vi "Write_CSV_date_time.vi"() -> ()   [LabVIEW 2015]
uses:
  <vilib>/Utility/file.llb/Write Delimited Spreadsheet (DBL).vi
  <vilib>/Utility/file.llb/Write To Spreadsheet File (string).vi
panel:
  in  "Values to Write":i32=20
  out "Array":string[](array[string])
  out "appended array":string[][](array[string])
  in  "# No Channel":i32=5
  in  "stop":bool
  in  "Header Info":string[][](table)=[["Test Name", "Operator", "UUT"], ["Voltage Test", "Nigel", "AAA123"]]
  in  "File Name":path=path "C:/Documents and Settings/husmith/Desktop/CSVdata.csv"
  in  "Channel Names":string[](array[string])=["Channel 1", "Channel 2", "Channel 3", "Channel 4", "Channel 5"]
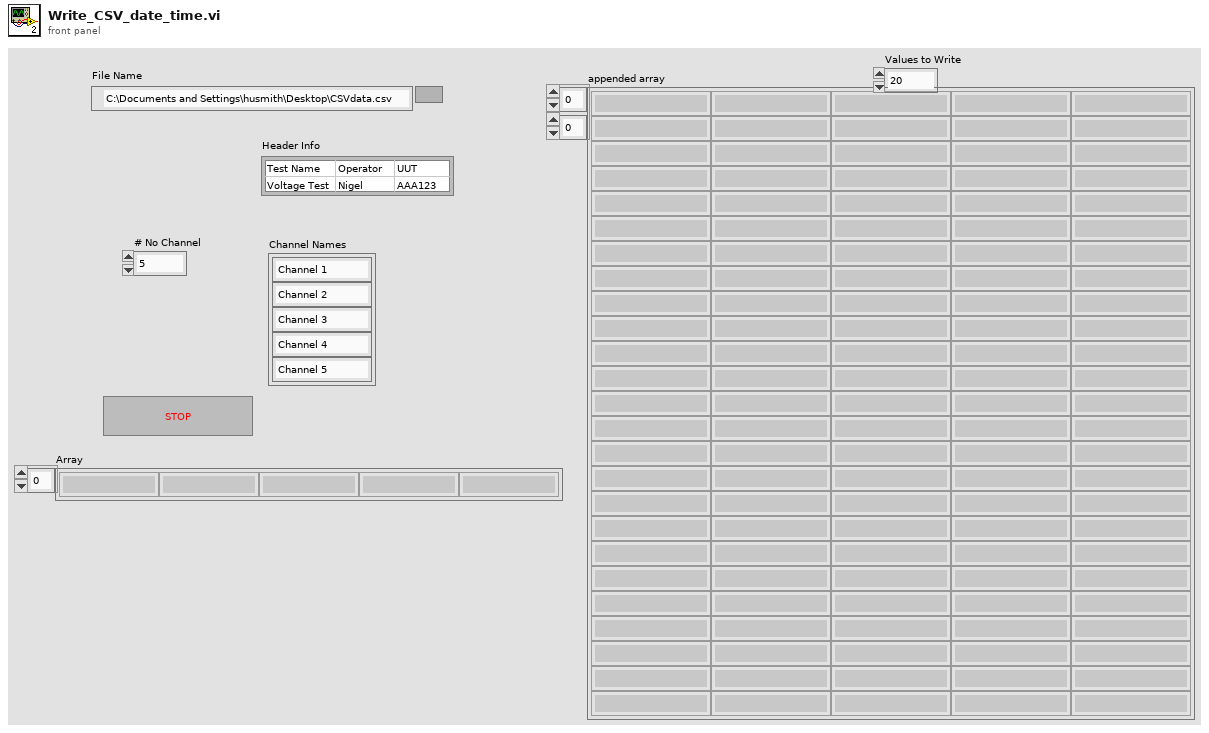
[diagram p1: front panel]
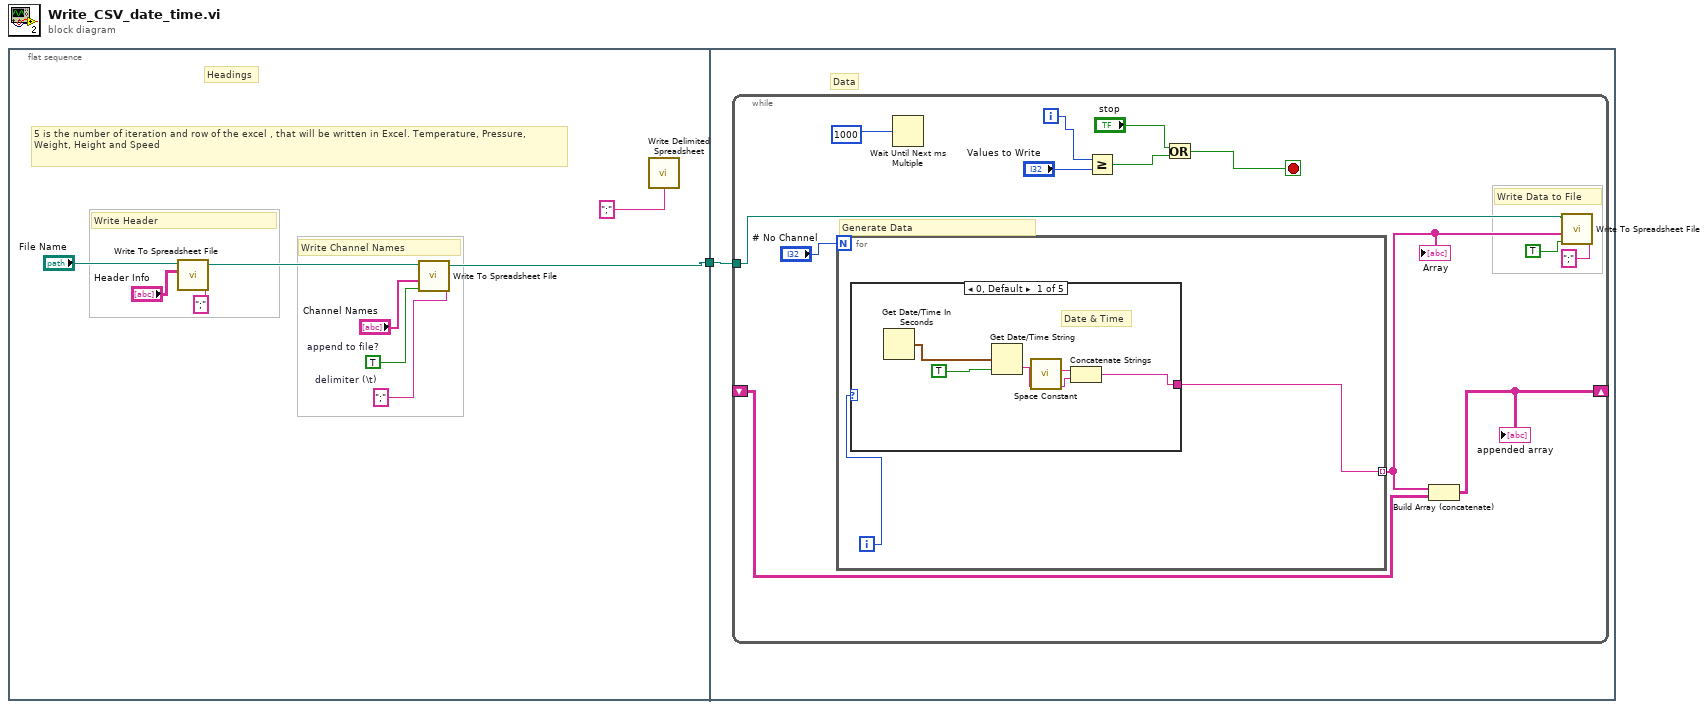
[diagram p0: block diagram]
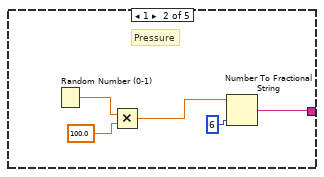
[diagram p2: hidden frame]
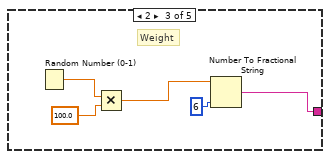
[diagram p3: hidden frame]
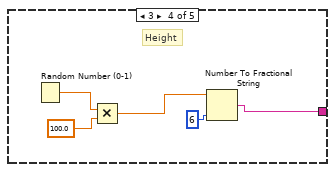
[diagram p4: hidden frame]
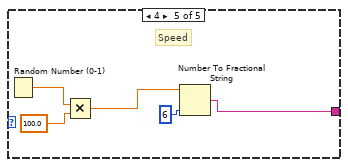
[diagram p5: hidden frame]
diagram:
  n1 = flat-sequence {
    tunnel: [w3] -> w1
    tunnel: w1 -> [w11]
    frame #0 {
      w7 = TRUE  # append to file?
      w8 = ";"  # delimiter (\t)
      # "Write Header"
      # "Write Channel Names"
      # "5 is the number of iteration and row of the excel , that will be written in Excel. Temperature, Pressure, Weight, Height and Speed"
      # "Headings"
      n2 = call-poly <vilib>:"Write To Spreadsheet File.vi"("delimiter (\\t)"=";" ("delimiter (\\t)"), "2D data"="Header Info", "file path (dialog if empty)"="File Name") -> ("new file path (Not A Path if cancelled)"=w9:path)  [unwired: 4 in, 1 out]
      n3 = call-poly <vilib>:"Write To Spreadsheet File.vi"("delimiter (\\t)"=w8, "append to file? (new file:F)"=w7, "1D data"="Channel Names", "file path (dialog if empty)"=w9) -> ("new file path (Not A Path if cancelled)"=w3:path)  [unwired: 3 in, 1 out]
    }
    frame #1 {
      # "Data"
      n4 = while {
        tunnel: w11 -> [w21]
        shift-right: [w17] -> _
        shift-left: _ -> [w19]
        i -> [w12]
        stop <- w14 stop-if-true
        # "Generate Data"
        # "Write Data to File"
        n5 = for {
          N: "# No Channel" -> [_]
          tunnel: [w25] -> w18 mode=indexing
          i -> [w26]
          n6 = case shown="0, Default" w26 {
            tunnel: [w30 w34 w37 w42 w47] -> w25
            frame 0, Default {
              # "Date & Time"
              n7 = Get Date/Time In Seconds() -> (seconds since 1Jan1904=w29:timestamp)
              n8 = Get Date/Time String(seconds (now)=w29, want seconds? (F)=TRUE) -> (time string=w28:string)  [unwired: 1 in, 1 out]
              n9 = call <vilib>:"Space Constant.vi"() -> ("String"=w27:string)
              n10 = Concatenate Strings(w27, w28) -> (w30:string)
            }
            frame 1 {
              # "Pressure"
              n11 = Random Number (0-1)() -> (number: 0 to 1=w36:dbl)
              n12 = Multiply(x=w36, y=100.0) -> (x*y=w33:dbl)
              n13 = Number To Fractional String(number=w33, precision (6)=i16 6) -> (F-format string=w34:string)  [unwired: 2 in]
            }
            frame 2 {
              # "Weight"
              n14 = Random Number (0-1)() -> (number: 0 to 1=w41:dbl)
              n15 = Multiply(x=w41, y=100.0) -> (x*y=w39:dbl)
              n16 = Number To Fractional String(number=w39, precision (6)=i16 6) -> (F-format string=w37:string)  [unwired: 2 in]
            }
            frame 3 {
              # "Height"
              n17 = Random Number (0-1)() -> (number: 0 to 1=w46:dbl)
              n18 = Multiply(x=w46, y=100.0) -> (x*y=w44:dbl)
              n19 = Number To Fractional String(number=w44, precision (6)=i16 6) -> (F-format string=w42:string)  [unwired: 2 in]
            }
            frame 4 {
              # "Speed"
              n20 = Random Number (0-1)() -> (number: 0 to 1=w51:dbl)
              n21 = Multiply(x=w51, y=100.0) -> (x*y=w49:dbl)
              n22 = Number To Fractional String(number=w49, precision (6)=i16 6) -> (F-format string=w47:string)  [unwired: 2 in]
            }
          }
        }
        "Array" <- w18
        n23 = Wait Until Next ms Multiple(millisecond multiple=u32 1000) -> ()  [unwired: 1 out]
        n24 = Greater Or Equal?(x=w12, y="Values to Write") -> (x >= y?=w15:bool)
        n25 = Or(x="stop", y=w15) -> (x .or. y?=w14:bool)
        n26 = Build Array (concatenate)(w18, w19) -> (w17:string[][])
        "appended array" <- w17
        n27 = call-poly <vilib>:"Write To Spreadsheet File.vi"("delimiter (\\t)"=";" ("delimiter (\\t)"), "append to file? (new file:F)"=TRUE, "1D data"=w18, "file path (dialog if empty)"=w21) -> ()  [unwired: 3 in, 2 out]
      }
    }
  }
  n28 = call-poly <vilib>:"Write Delimited Spreadsheet.vi"("delimiter (\\t)"=";" ("delimiter (\\t)")) -> ()  [unwired: 13 in, 2 out]
